vi "简易版温湿度监控.vi"() -> ()   [LabVIEW 2020]
uses:
  <vilib>/Instr/_visa.llb/VISA Configure Serial Port (Instr).vi
panel:
  out "String 11":string="手控开关"
  out "温度":dbl
  out "湿度":dbl
  out "String 10":string="控制方式"
  out "String 9":string="手动"
  out "String 8":string="自动"
  in  "控制开关":bool
  out "String 6":string="指示灯"
  out "String 7":string="手控开关"
  in  "风扇":bool
  in  "加湿器":bool
  out "风扇":bool
  out "String 2":string="监控板"
  out "加湿器":bool
  in  "停止":bool
  out "String 3":string="温湿度监控系统"
  out "String":string="采集板"
  in  "Tab Control":enum32{"通讯设置", "数据操作", "温度采集", "湿度采集"}(tab)
  in  "确定":bool
  in  "修改":bool
  in  "发送":string
  out "读取缓冲区":string
  in  "串口选择":refnum<visa-resource-name>
  in  "保存":bool
  out "字节1":string
  out "字节2":string
  out "字节3":string
  out "字节4":string
  out "1":u32
  out "2":u32
  out "3":u32
  out "字符串":string="十进制"
  out "字符串 2":string="十六进制"
  out "字节5":string
  out "5":u32
  out "4":u32
  out "Waveform Chart":u32(graph)
  out "String 4":string="温度采集"
  out "Thermometer":dbl(slide) scale=0.0..100.0
  out "Waveform Chart 2":u32(graph)
  out "String 5":string="湿度采集"
  out "Gauge":dbl(knob) scale=0.0..100.0
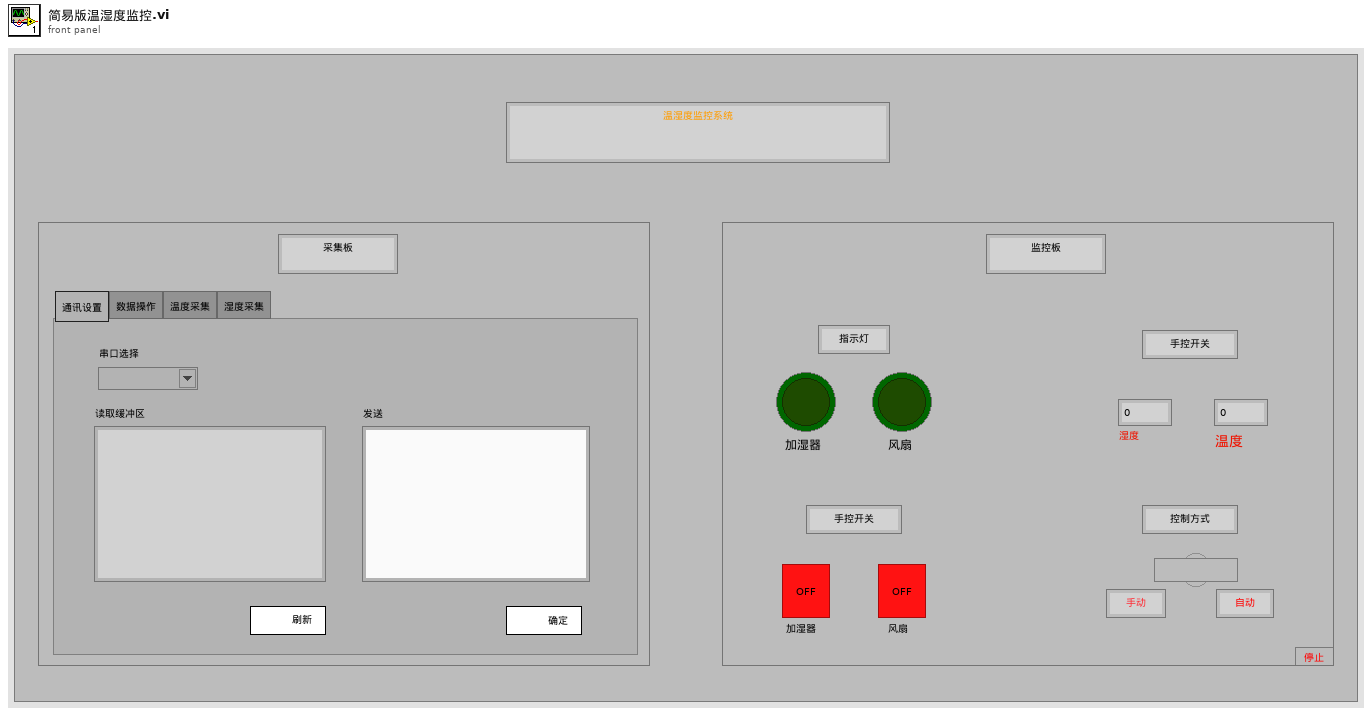
[diagram p1: front panel]
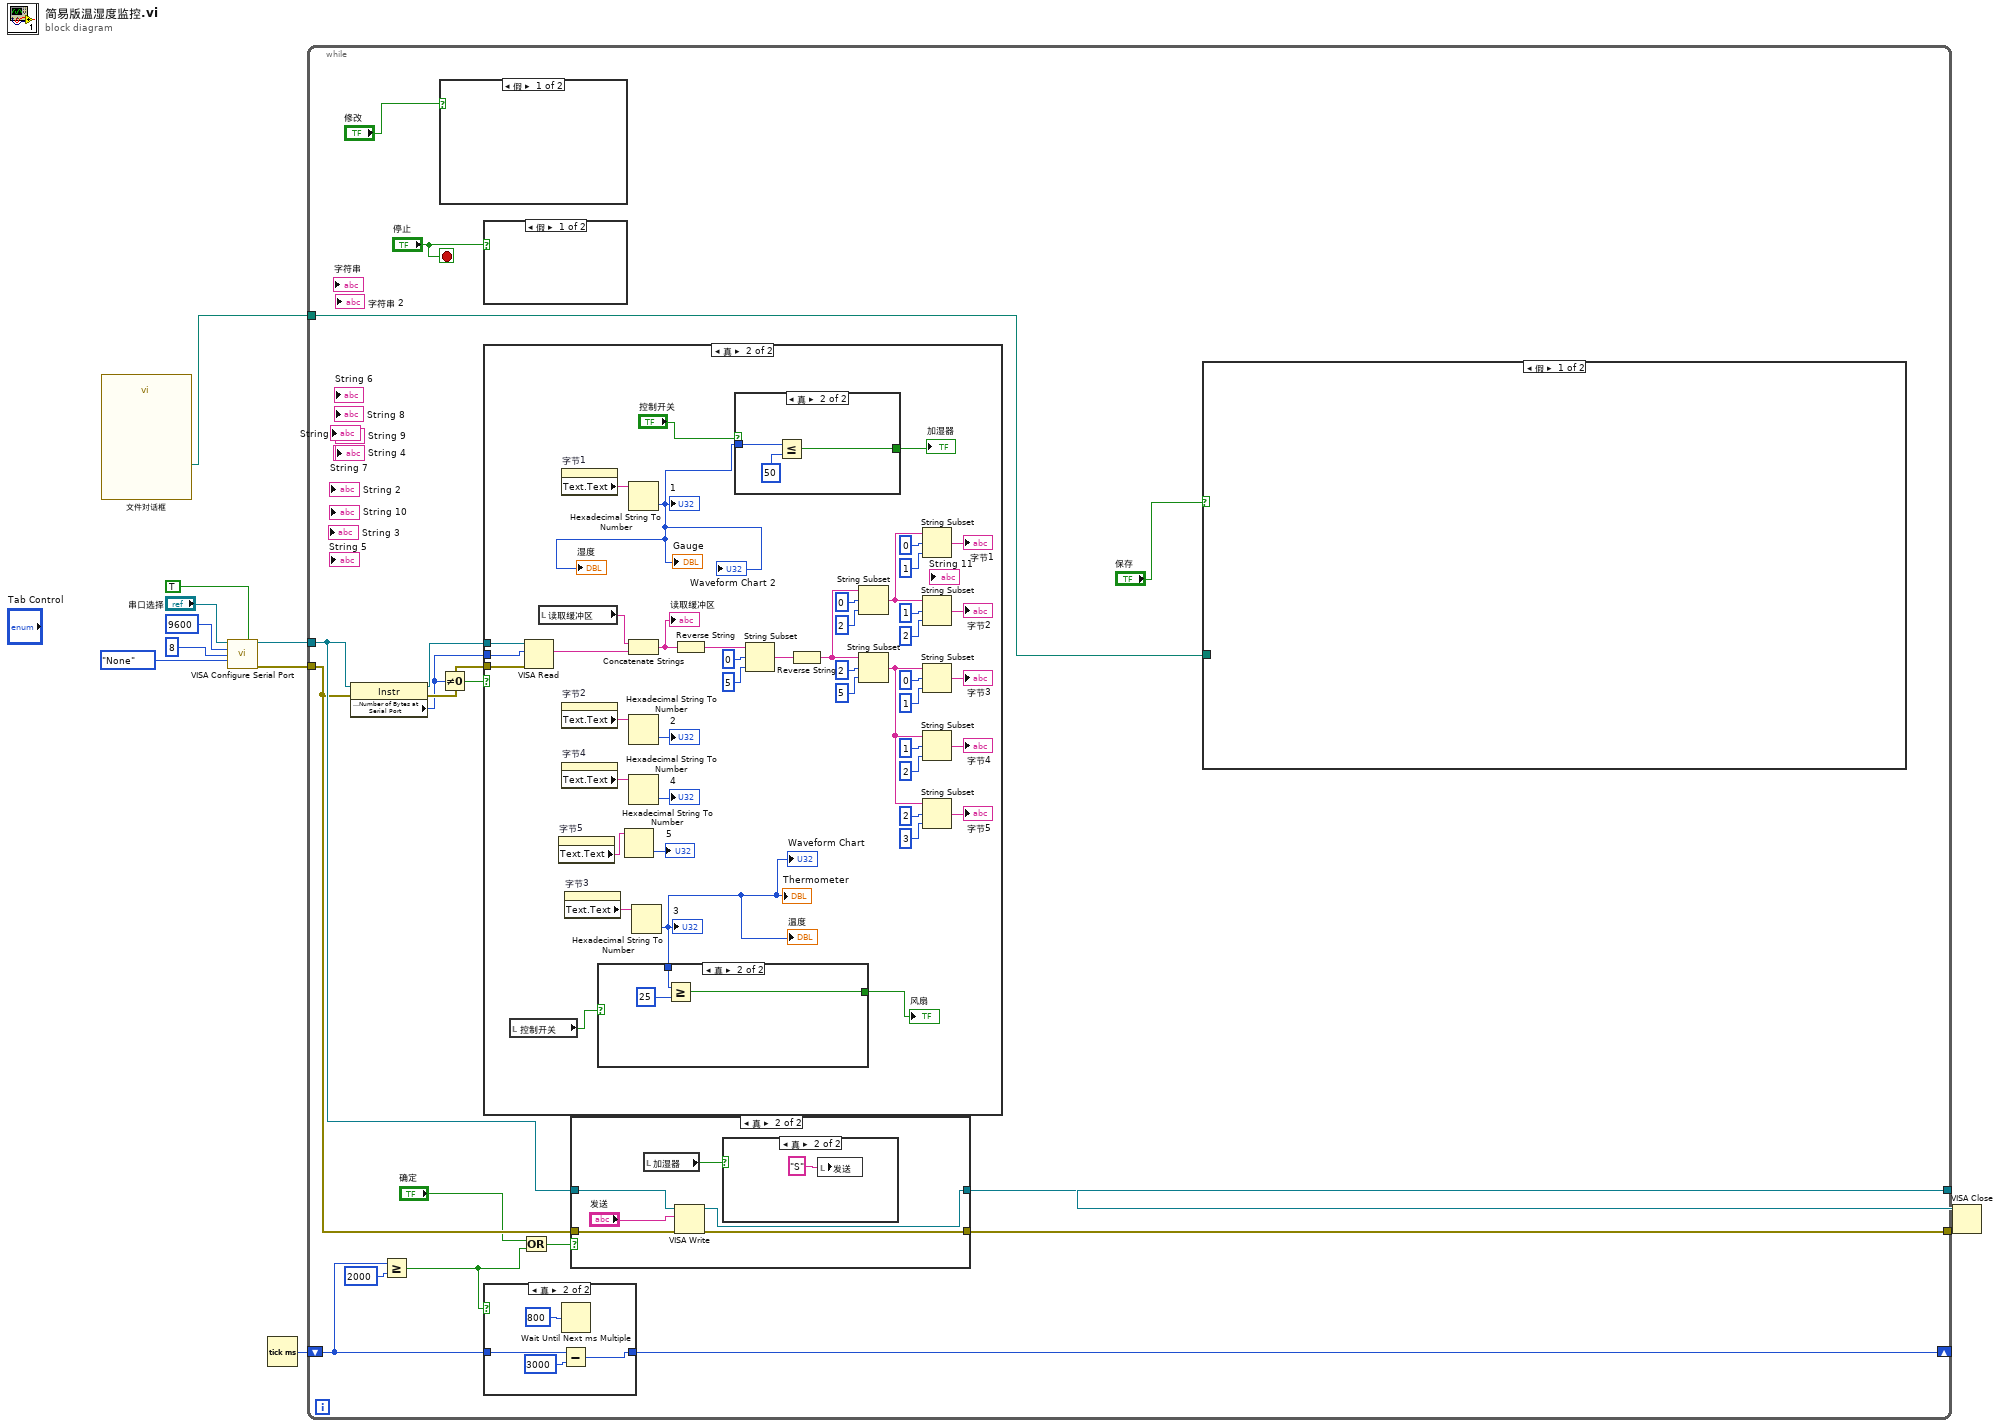
[diagram p0: block diagram]
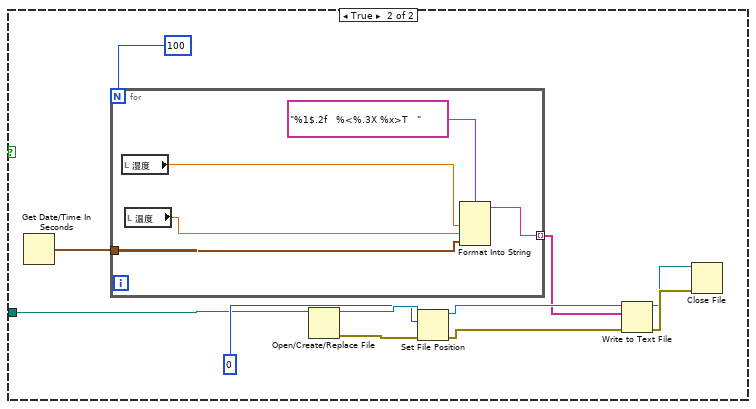
[diagram p2: hidden frame]
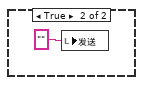
[diagram p3: hidden frame]
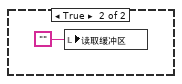
[diagram p5: hidden frame]
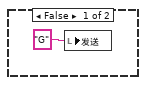
[diagram p7: hidden frame]
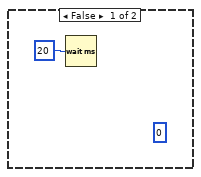
[diagram p8: hidden frame]
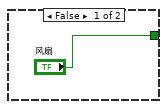
[diagram p9: hidden frame]
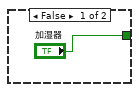
[diagram p10: hidden frame]
diagram:
  n1 = call "文件对话框"() -> ("selected path"=w1:path)  [unwired: 12 in, 3 out]
  n2 = call-poly "VISA Configure Serial Port"("VISA resource name"="串口选择", "Enable Termination\nChar (T)"=TRUE ("Enable Termination\nChar (T)"), "baud rate (9600)"=u32 9600, "data bits (8)"=u16 8, "parity (0:none)"=enum16{"None", "Odd", "Even", "Mark", "Space"}."None") -> ("VISA resource name out"=w6:refnum<visa-resource-name>, "error out"=w5:errorcluster)  [unwired: 9 in]
  n3 = Tick Count (ms)() -> (millisecond timer value=w2:u32)
  n4 = while {
    tunnel: w6 -> [w25]
    tunnel: w5 -> [w24]
    tunnel: [w23] -> w4
    tunnel: [w22] -> w3
    shift-right: [w18] -> _
    shift-left: w2 -> [w17]
    tunnel: w1 -> [w12]
    stop <- "停止" stop-if-true
    n5 = property class="Instr"(reference=w25, error in=w24) -> (reference out=w29:refnum<visa-resource-name>, error out=w28:errorcluster, "Serial Settings:Number of Bytes at Serial Port"=w26:u32)
    n6 = Greater Or Equal?(x=w17, y=u32 2000) -> (x >= y?=w20:bool)
    n7 = case shown="假" "修改" {
      frame False {
      }
      frame True {
        n8 = local write "读取缓冲区"("") -> ()
      }
    }
    n9 = Not Equal To 0?(x=w26) -> (x != 0?=w27:bool)
    n10 = case shown="假" "停止" {
      frame False {
      }
      frame True {
        n11 = local write "发送"("") -> ()
      }
    }
    n12 = case shown="真" w27 {
      tunnel: w29 -> [_ w109]
      tunnel: w28 -> [_ w108]
      tunnel: w26 -> [_ w107]
      frame False {
        (unwired) u32 0
        n13 = Wait (ms)(milliseconds to wait=u32 20 ("等待时间（毫秒）")) -> ()  [unwired: 1 out]
      }
      frame True {
        n14 = local read "控制开关"() -> (w66:bool)
        n15 = VISA Read(VISA resource name=w109, byte count=w107, error in (no error)=w108) -> (read buffer=w105:string)  [unwired: 3 out]
        n16 = local read "读取缓冲区"() -> (w106:string)
        n17 = property on="字节5" class="Str"() -> ("Text.Text"=w73:string)  [unwired: 2 in, 2 out]
        n18 = property on="字节1" class="Str"() -> ("Text.Text"=w82:string)  [unwired: 2 in, 2 out]
        n19 = property on="字节2" class="Str"() -> ("Text.Text"=w80:string)  [unwired: 2 in, 2 out]
        n20 = property on="字节4" class="Str"() -> ("Text.Text"=w71:string)  [unwired: 2 in, 2 out]
        n21 = property on="字节3" class="Str"() -> ("Text.Text"=w81:string)  [unwired: 2 in, 2 out]
        n22 = Hexadecimal String To Number(string=w73) -> (number=→"5":u32)  [unwired: 2 in, 1 out]
        n23 = Hexadecimal String To Number(string=w82) -> (number=w64:u32)  [unwired: 2 in, 1 out]
        "1" <- w64
        "Gauge" <- w64
        "Waveform Chart 2" <- w64
        "湿度" <- w64
        n24 = Concatenate Strings(w106, w105) -> (w79:string)
        "读取缓冲区" <- w79
        n25 = Hexadecimal String To Number(string=w80) -> (number=→"2":u32)  [unwired: 2 in, 1 out]
        n26 = Hexadecimal String To Number(string=w71) -> (number=→"4":u32)  [unwired: 2 in, 1 out]
        n27 = Hexadecimal String To Number(string=w81) -> (number=w67:u32)  [unwired: 2 in, 1 out]
        "3" <- w67
        "Thermometer" <- w67
        "Waveform Chart" <- w67
        "温度" <- w67
        n28 = case shown="真" w66 {
          tunnel: w67 -> [_ w113]
          tunnel: ["风扇" w111] -> w65
          frame False {
          }
          frame True {
            n29 = Greater Or Equal?(x=w113, y=u32 25) -> (x >= y?=w111:bool)
          }
        }
        "风扇" <- w65
        n30 = Reverse String(1:w79) -> (0:w102:string)
        n31 = case shown="真" "控制开关" {
          tunnel: w64 -> [_ w116]
          tunnel: ["加湿器" w115] -> w68
          frame False {
          }
          frame True {
            n32 = Less Or Equal?(x=w116, y=u32 50) -> (x <= y?=w115:bool)
          }
        }
        "加湿器" <- w68
        n33 = String Subset(string=w102, offset (0)=0 ("偏移量(0)"), length (rest)=5 ("长度（剩余）")) -> (substring=w101:string)
        n34 = Reverse String(1:w101) -> (0:w91:string)
        n35 = String Subset(string=w91, offset (0)=0 ("偏移量(0)"), length (rest)=2 ("长度（剩余）")) -> (substring=w92:string)
        n36 = String Subset(string=w91, offset (0)=2 ("偏移量(0)"), length (rest)=5 ("长度（剩余）")) -> (substring=w77:string)
        n37 = String Subset(string=w92, offset (0)=0 ("偏移量(0)"), length (rest)=1 ("长度（剩余）")) -> (substring=→"字节1":string)
        n38 = String Subset(string=w92, offset (0)=1 ("偏移量(0)"), length (rest)=2 ("长度（剩余）")) -> (substring=→"字节2":string)
        n39 = String Subset(string=w77, offset (0)=0 ("偏移量(0)"), length (rest)=1 ("长度（剩余）")) -> (substring=→"字节3":string)
        n40 = String Subset(string=w77, offset (0)=1 ("偏移量(0)"), length (rest)=2 ("长度（剩余）")) -> (substring=→"字节4":string)
        n41 = String Subset(string=w77, offset (0)=2, length (rest)=3 ("length (rest)")) -> (substring=→"字节5":string)
      }
    }
    n42 = case shown="真" w20 {
      tunnel: [w47 w50] -> w18
      tunnel: w17 -> [w47 w48]
      frame False {
      }
      frame True {
        n43 = Wait Until Next ms Multiple(millisecond multiple=u32 800 ("毫秒倍数")) -> ()  [unwired: 1 out]
        n44 = Subtract(x=w48, y=u32 3000) -> (x-y=w50:u32)
      }
    }
    n45 = Or(x="确定", y=w20) -> (x .or. y?=w19:bool)
    n46 = case shown="真" w19 {
      tunnel: [w54 w60] -> w23
      tunnel: [w53 w59] -> w22
      tunnel: w25 -> [w54 w58]
      tunnel: w24 -> [w53 w57]
      frame False {
      }
      frame True {
        n47 = local read "加湿器"() -> (w55:bool)
        n48 = VISA Write(VISA resource name=w58, write buffer="发送", error in (no error)=w57) -> (VISA resource name out=w60:refnum<visa-resource-name>, error out=w59:errorcluster)  [unwired: 1 out]
        n49 = case shown="真" w55 {
          frame False {
            n50 = local write "发送"("G") -> ()
          }
          frame True {
            n51 = local write "发送"("S") -> ()
          }
        }
      }
    }
    n52 = case shown="假" "保存" {
      tunnel: w12 -> [_ w30]
      frame False {
      }
      frame True {
        n53 = Get Date/Time In Seconds() -> (seconds since 1Jan1904=w40:timestamp)
        n54 = for {
          N: 100 -> [_]
          tunnel: [w44] -> w31 mode=indexing
          tunnel: w40 -> [w41]
          n55 = local read "湿度"() -> (w43:dbl)
          n56 = local read "温度"() -> (w42:dbl)
          n57 = Format Into String(format string="%1$.2f   %<%.3X %x>T   " ("格式字符串"), w43, w42, w41) -> (resulting string=w44:string)  [unwired: 2 in, 1 out]
        }
        n58 = Open/Create/Replace File(file path (use dialog)=w30) -> (refnum out=w34:refnum<file>, error out=w37:errorcluster)  [unwired: 5 in, 1 out]
        n59 = Set File Position(offset (in bytes) (0)=i64 0 ("偏移量（字节）（0）"), refnum=w34, error in=w37) -> (refnum out=w38:refnum<file>, error out=w39:errorcluster)  [unwired: 1 in]
        n60 = Write to Text File(file (use dialog)=w38, text=w31, error in=w39) -> (refnum out=w35:refnum<file>, error out=w36:errorcluster)  [unwired: 1 in, 1 out]
        n61 = Close File(refnum=w35, error in=w36) -> ()  [unwired: 2 out]
      }
    }
  }
  n62 = VISA Close(VISA resource name=w4, error in (no error)=w3) -> ()  [unwired: 1 out]
